vi "Interpolate Parameter.vi"(8 "error in (no error)":errorcluster, 9 "Fake Point":dbl, 10 "Parameter-array":dbl[](array[numeric]) format="%.2p", 11 "XY-data":cluster{"X-array":dbl[], "Y-array":dbl[]}[](array[cluster]) {"Y-array" format="%.2p"; "X-array" format="%.2p"}) -> (0 "error out":errorcluster, 2 "Interpolated Parameter-array":dbl[](array[numeric]), 3 "Interpolated XY-data out":cluster{"X-array":dbl[], "Y-array":dbl[]}[](array[cluster]) {"Y-array" format="%.2p"; "X-array" format="%.2p"})   [LabVIEW 2019, in "xy_utilities.lvlib"]
doc: "Interpolate the input <b>XY-data</b> along the <b>Parameter-array</b> axis."
uses:
  xy_utilities.lvlib
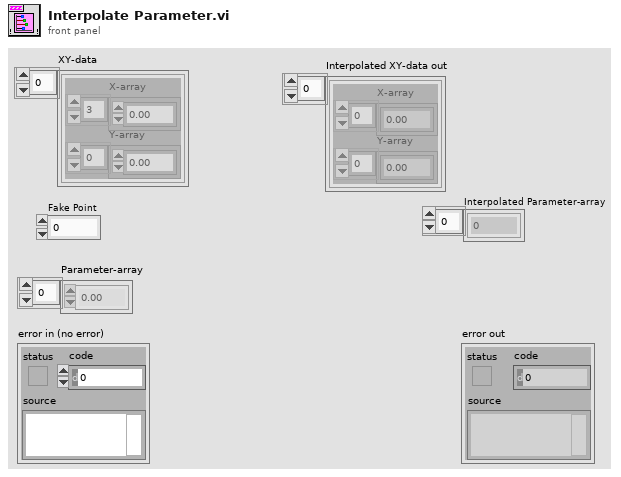
[diagram p1: front panel]
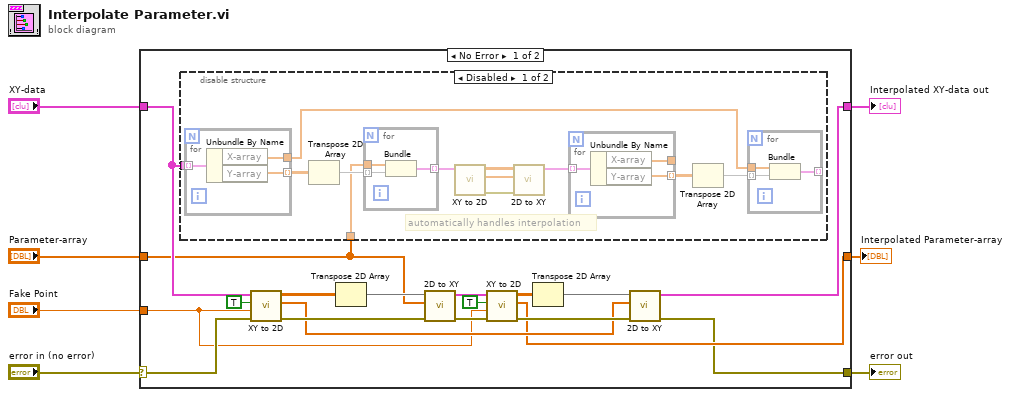
[diagram p0: block diagram]
diagram:
  n1 = case shown="No Error" "error in (no error)" {
    selector: "error in (no error)" -> [w16 w52]
    tunnel: "XY-data" -> [w17 w51]
    tunnel: [w13 w51] -> w5
    tunnel: [w11 w52] -> w4
    tunnel: "Parameter-array" -> [w15 w50]
    tunnel: [w12 w50] -> w2
    tunnel: "Fake Point" -> [w10 _]
    frame No Error {
      n2 = disable-structure shown="Disabled" {
        disable-tunnel: w17 -> [w27 _]
        disable-tunnel: w15 -> [w26 _]
        frame Disabled {
          # "automatically handles interpolation"
          n3 = for {
            tunnel: w27 -> [w49] mode=indexing
            tunnel: [w48] -> w37 mode=indexing
            tunnel: [w47] -> w33
            n4 = Unbundle By Name(w49) -> ("X-array"=w47:dbl[], "Y-array"=w48:dbl[])
          }
          n5 = Transpose 2D Array(2D array=w37) -> (transposed array=w36:dbl[][])
          n6 = for {
            tunnel: w36 -> [w46] mode=indexing
            tunnel: w26 -> [w45]
            tunnel: [w44] -> w29 mode=indexing
            n7 = Bundle("Parameter-array"=w45, w46) -> (w44:cluster{"Parameter-array":dbl[], dbl[]})  [unwired: 1 in]
          }
          n8 = call "XY to 2D.vi"("XY-data"=w29) -> ("error out"=w30:errorcluster, "X Array"=w31:dbl[], "2D Y Array"=w32:dbl[][])  [unwired: 7 in, 1 out]
          n9 = call "2D to XY.vi"("error in (no error)"=w30, "X Array"=w31, "2D Y Array"=w32) -> ("XY-data out"=w28:cluster{"X-array":dbl[], "Y-array":dbl[]}[])  [unwired: 7 in, 1 out]
          n10 = for {
            tunnel: w28 -> [w43] mode=indexing
            tunnel: [w42] -> w34 mode=indexing
            tunnel: [w41] -> _
            n11 = Unbundle By Name(w43) -> ("X-array"=w41:dbl[], "Y-array"=w42:dbl[])
          }
          n12 = Transpose 2D Array(2D array=w34) -> (transposed array=w35:dbl[][])
          n13 = for {
            tunnel: w35 -> [w40] mode=indexing
            tunnel: w33 -> [w39]
            tunnel: [w38] -> _ mode=indexing
            n14 = Bundle("X-array"=w39, w40) -> (w38:cluster{"X-array":dbl[], dbl[]})  [unwired: 1 in]
          }
        }
        frame Enabled {
        }
      }
      n15 = call "XY to 2D.vi"("error in (no error)"=w16, "Fake Point"=w10, "Interpolate [T]"=TRUE, "XY-data"=w17) -> ("error out"=w25:errorcluster, "X Array"=w14:dbl[], "2D Y Array"=w24:dbl[][])  [unwired: 4 in, 1 out]
      n16 = Transpose 2D Array(2D array=w24) -> (transposed array=w23:dbl[][])
      n17 = call "2D to XY.vi"("error in (no error)"=w25, "X Array"=w15, "2D Y Array"=w23) -> ("error out"=w19:errorcluster, "XY-data out"=w22:cluster{"X-array":dbl[], "Y-array":dbl[]}[])  [unwired: 7 in]
      n18 = call "XY to 2D.vi"("error in (no error)"=w19, "Fake Point"=w10, "Interpolate [T]"=TRUE, "XY-data"=w22) -> ("error out"=w21:errorcluster, "X Array"=w12:dbl[], "2D Y Array"=w18:dbl[][])  [unwired: 4 in, 1 out]
      n19 = Transpose 2D Array(2D array=w18) -> (transposed array=w20:dbl[][])
      n20 = call "2D to XY.vi"("error in (no error)"=w21, "X Array"=w14, "2D Y Array"=w20) -> ("error out"=w11:errorcluster, "XY-data out"=w13:cluster{"X-array":dbl[], "Y-array":dbl[]}[])  [unwired: 7 in]
    }
    frame Error {
    }
  }
  "error out" <- w4
  "Interpolated XY-data out" <- w5
  "Interpolated Parameter-array" <- w2
